vi "ReadAdsTimeout.vi"(8 "error in (no error)":errorcluster, 11 "AdsNET in":refnum<class "AdsNET.lvclass">) -> (0 "error out":errorcluster, 2 "Timeout":i32, 3 "AdsNET out":refnum<class "AdsNET.lvclass">)   [LabVIEW 2016, in "TCatAdsNet.lvlib" / "AdsNET.lvclass"]
doc: "Read the timeout for the ADS communication. Unit is in ms."
uses:
  AdsNET.lvclass
  AdsNET.lvclass/AdsNET.ctl
  C:/Users/Maurizio/Projects/twincat-lv-ads-library/TCatAdsNet Library/TwinCAT.Ads.dll
  TwinCAT.Ads.dll
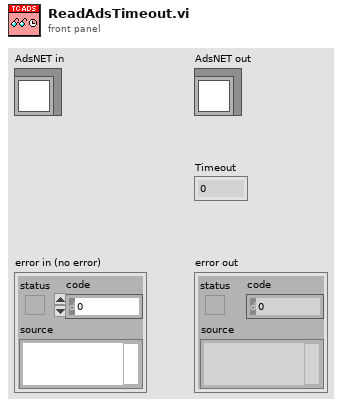
[diagram p1: front panel]
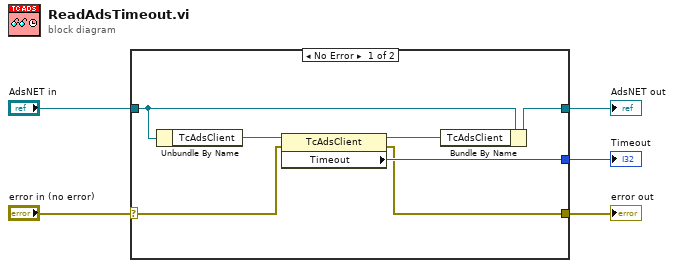
[diagram p0: block diagram]
diagram:
  n1 = case shown="No Error" "error in (no error)" {
    selector: "error in (no error)" -> [w7 w14]
    tunnel: [w6 w14] -> w4
    tunnel: [w9 w13] -> w2
    tunnel: "AdsNET in" -> [w12 w13]
    tunnel: [w10 _] -> w1
    frame No Error {
      n2 = Unbundle By Name(w12) -> ("TcAdsClient"=w11:refnum<k24>)
      n3 = property class="TcAdsClient"(reference=w11, error in=w7) -> (reference out=w8:refnum<k24>, error out=w6:errorcluster, "Timeout"=w10:i32)
      n4 = Bundle By Name(cluster=w12, "TcAdsClient"=w8) -> (w9:refnum<class "AdsNET.lvclass">)
    }
    frame Error {
    }
  }
  "error out" <- w4
  "AdsNET out" <- w2
  "Timeout" <- w1
